vi "Equal.vi"() -> ()   [LabVIEW 2017, in "Transparent Assertions.Tests.lvlib" / "Assert Less Than.lvlib"]
uses:
  Assert Less Than.lvlib
  src/Transparent Assertions/Transparent Assertions.lvlib
panel:
  out "error out":errorcluster
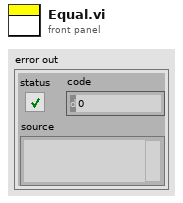
[diagram p1: front panel]
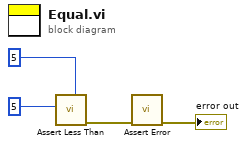
[diagram p0: block diagram]
diagram:
  n1 = call "Assert Less Than.vi"("Expected"=5, "Actual"=5) -> ("error out"=w2:errorcluster)  [unwired: 9 in]
  n2 = call "Assert Error.vi"("error in (no error)"=w2) -> ("error out"=→"error out":errorcluster)  [unwired: 10 in]
